vi "array template.vi"() -> ()   [LabVIEW 2012]
uses:
  <vilib>/Utility/VariantDataType/VariantType.lvlib
panel:
  out "Array Size":i32[](array[numeric])
  in  "Array":dbl[](array[numeric])
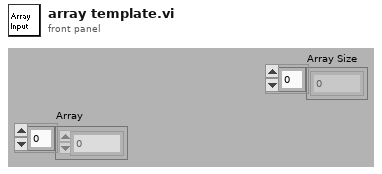
[diagram p1: front panel]
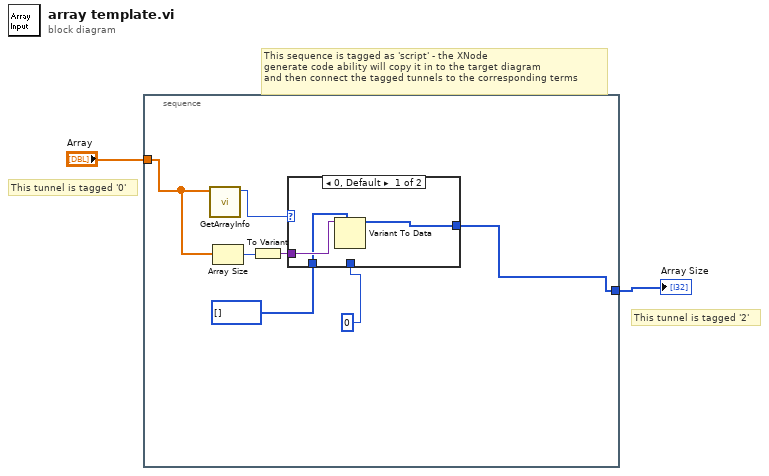
[diagram p0: block diagram]
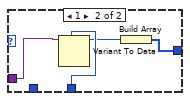
[diagram p2: hidden frame]
diagram:
  # "This tunnel is tagged '2'"
  # "This tunnel is tagged '0'"
  # "This sequence is tagged as 'script' - the XNode \ngenerate code ability will copy it in to the target diagram\nand then connect the tagged tunnels to the corresponding terms"
  n1 = stacked-sequence {
    tunnel: "Array" -> [w9]
    tunnel: [w3] -> w1
    frame #0 {
      n2 = call <vilib>:"GetArrayInfo.vi"("Variant"=w9) -> ("NDims"=w6:i32)  [unwired: 1 in, 9 out]
      n3 = Array Size(array=w9) -> (size(s)=w8:i32)
      n4 = To Variant(anything=w8) -> (Variant=w7:variant)
      n5 = case shown="0, Default" w6 {
        tunnel: w7 -> [w12 w16]
        tunnel: i32[] [] -> [w11 _]
        tunnel: 0 -> [_ w15]
        tunnel: [w10 w13] -> w3
        frame 0, Default {
          n6 = Variant To Data(type=w11, Variant=w12) -> (data=w10:i32[])  [unwired: 1 in, 1 out]
        }
        frame 1 {
          n7 = Variant To Data(type=w15, Variant=w16) -> (data=w14:i32)  [unwired: 1 in, 1 out]
          n8 = Build Array(w14) -> (w13:i32[])
        }
      }
    }
  }
  "Array Size" <- w1
